vi "Chrg_Dschrg.vi"(3 "Strain Offset":dbl, 4 "PS VISA in":refnum<visa-resource-name>, 5 "PS error in":errorcluster caption="PS error in (no error)", 6 "CyclePath":path=path "C:/Users/ga11/Desktop/VI/results/3PtestCharge.lvm" caption="Filename", 7 "Battery Type":T1(ring), 8 "Charge/discharge":enum8{"Charge", "Discharge"}(ring), 9 "Charge/Discharge Voltage Setpoint":dbl format="%#.6g", 11 "Current Setpoint":dbl format="%#.6g", 13 "Current Cutoff":dbl) -> (14 "PS VISA out":refnum<visa-resource-name>, 16 "Boolean":bool, 19 "PS error out":errorcluster)   [LabVIEW 2020]
uses:
  Drivers-IT-M3400/IT-M3400.lvlib
  <vilib>/Utility/TradDaqScaling.llb/Convert Strain Gauge Reading (scaler).vi
panel:
  out "Read Current(A)":dbl format="%.2g"
  out "Read Voltage(V)":dbl format="%.2g"
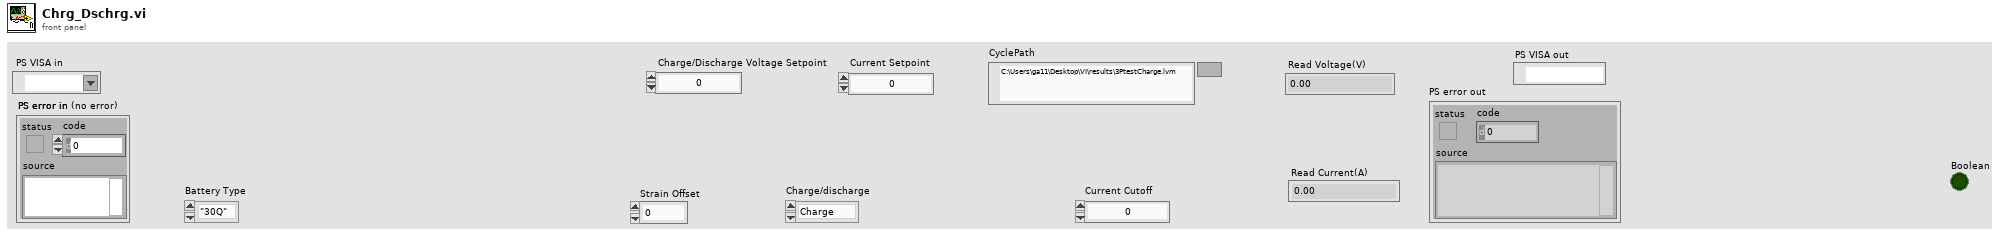
[diagram p1: front panel]
types:
  T1 = enum16{"\"30Q\"", "\"40T\"", "\"2P30Q\"", "\"3P30Q\"", "\"Nissan Leaf\""}
  T2 = cluster{"Baud Rate":u32, "Parity":u16, "Data Bits":u16, "Stop Bits":u16, "Flow Control":u16}
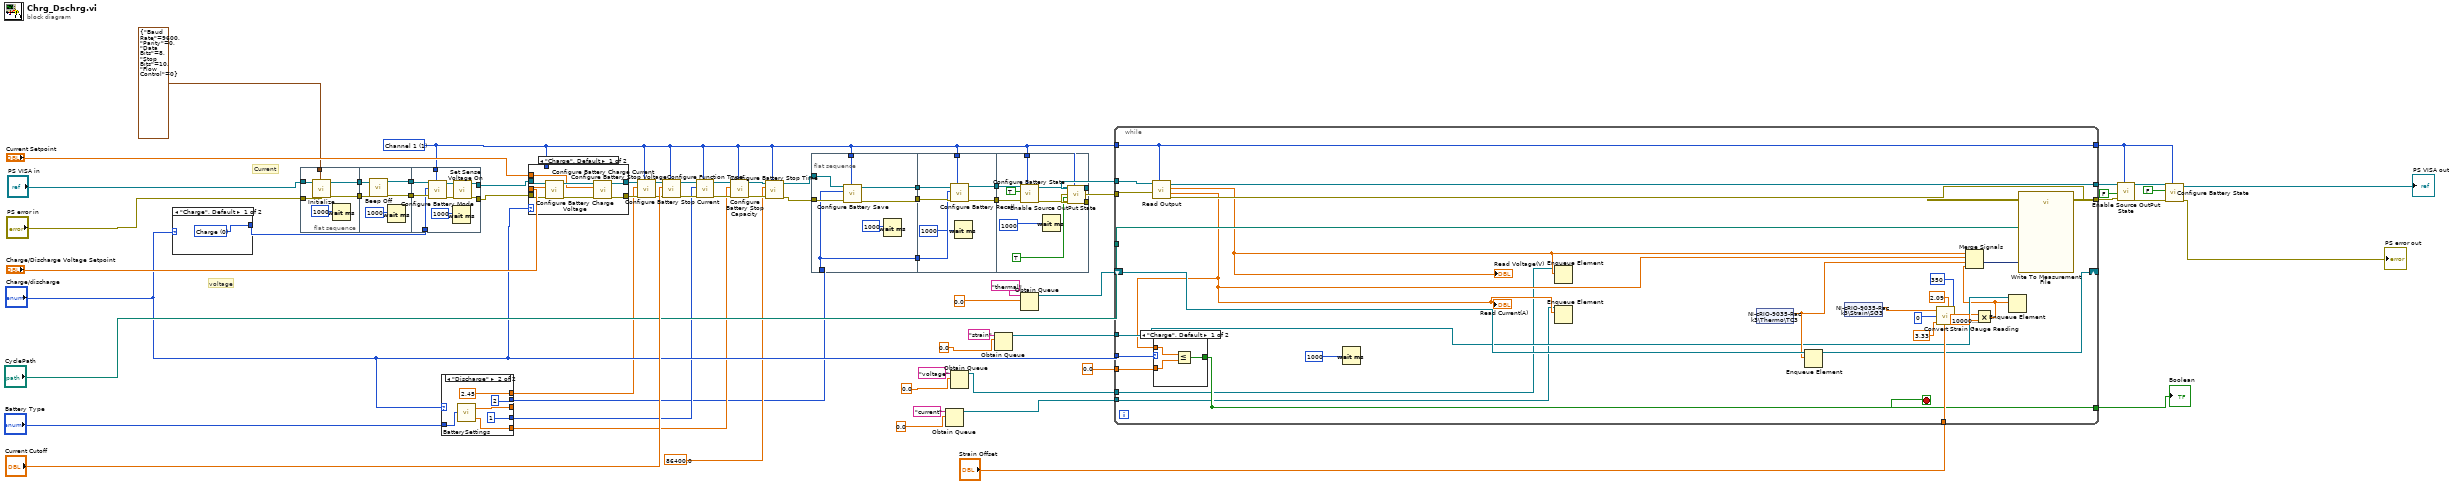
[diagram p0: block diagram]
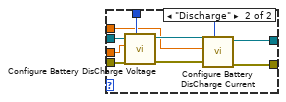
[diagram p2: hidden frame]
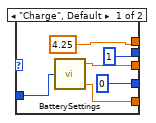
[diagram p3: hidden frame]
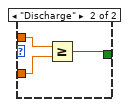
[diagram p4: hidden frame]
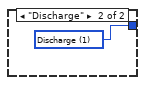
[diagram p5: hidden frame]
diagram:
  w3 = 1 items=["Channel 1"=1, "Channel 2"=2, "Channel 3"=3, "Channel 4"=4, "Channel 5"=5, "Channel 6"=6, "Channel 7"=7, "Channel 8"=8, "Channel 8"=9, "Channel 10"=10, "Channel 11"=11, "Channel 12"=12, "Channel 13"=13, "Channel 14"=14, "Channel 15"=15, "Channel 16"=16] ("Channel")
  # "voltage"
  # "Current"
  n1 = case shown="\"Charge\", Default" "Charge/discharge" {
    tunnel: [w66 w67] -> w6
    frame "Charge", Default {
      w66 = u8 0 items=["Charge", "Discharge"] ("Battery Mode")
    }
    frame "Discharge" {
      w67 = u8 1 items=["Charge", "Discharge"] ("Battery Mode")
    }
  }
  n2 = flat-sequence {
    tunnel: T2 {"Baud Rate"=9600, "Parity"=0, "Data Bits"=8, "Stop Bits"=10, "Flow Control"=0} ("Serial Configuration") -> [w73]
    tunnel: "PS error in" -> [w72]
    tunnel: "PS VISA in" -> [w71]
    tunnel: [w69] -> w11
    tunnel: [w68] -> w10
    tunnel: [w77] -> w9
    tunnel: [w76] -> w8
    tunnel: w11 -> [w75]
    tunnel: w10 -> [w74]
    tunnel: w9 -> [w85]
    tunnel: w8 -> [w86]
    tunnel: w3 -> [w87]
    tunnel: [w80] -> w1
    tunnel: [w81] -> w2
    tunnel: w6 -> [w79]
    frame #0 {
      n3 = call "Initialize.vi"("Serial Configuration"=w73, "error in"=w72, "VISA resource name"=w71) -> ("error out"=w68:errorcluster, "VISA resource name out"=w69:refnum<visa-resource-name>)  [unwired: 7 in]
      n4 = Wait (ms)(milliseconds to wait=1000) -> ()  [unwired: 1 out]
    }
    frame #1 {
      n5 = call "Beep Off.vi"("error in"=w74, "VISA resource name"=w75) -> ("error out"=w76:errorcluster, "VISA resource name out"=w77:refnum<visa-resource-name>)  [unwired: 8 in]
      n6 = Wait (ms)(milliseconds to wait=1000) -> ()  [unwired: 1 out]
    }
    frame #2 {
      n7 = call "Configure Battery Mode.vi"("Channel"=w87, "error in"=w86, "Battery Mode"=w79, "VISA resource name"=w85) -> ("error out"=w82:errorcluster, "VISA resource name out"=w83:refnum<visa-resource-name>)  [unwired: 6 in]
      n8 = Wait (ms)(milliseconds to wait=1000) -> ()  [unwired: 1 out]
      n9 = call "Set Sense Voltage On.vi"("error in"=w82, "VISA resource name"=w83) -> ("error out"=w80:errorcluster, "VISA resource name out"=w81:refnum<visa-resource-name>)  [unwired: 8 in]
    }
  }
  n10 = case shown="\"Discharge\"" "Charge/discharge" {
    tunnel: "Battery Type" -> [w93 w99]
    tunnel: [w92 w97] -> _
    tunnel: [u8 0 ("File") u8 1 ("File")] -> w29
    tunnel: [u8 1 ("File") u8 2 ("File")] -> w27
    tunnel: [w89 w95] -> w28
    tunnel: [4.25 2.45] -> w26
    frame "Charge", Default {
      n11 = call "BatterySettings.vi"("Battery Type"=w93) -> ("RatedCapacity (Ah)"=w89:dbl, "Max Voltage (V)"=w92:dbl)  [unwired: 2 in, 1 out]
    }
    frame "Discharge" {
      n12 = call "BatterySettings.vi"("Battery Type"=w99) -> ("RatedCapacity (Ah)"=w95:dbl, "Min Voltage (V)"=w97:dbl)  [unwired: 2 in, 1 out]
    }
  }
  n13 = case shown="\"Charge\", Default" "Charge/discharge" {
    tunnel: w2 -> [w107 w116]
    tunnel: w1 -> [w106 w115]
    tunnel: [w101 w112] -> w44
    tunnel: [w100 w111] -> w43
    tunnel: w3 -> [_ w110]
    tunnel: "Charge/Discharge Voltage Setpoint" -> [w103 w109]
    tunnel: "Current Setpoint" -> [w102 w108]
    frame "Charge", Default {
      n14 = call "Configure Battery Charge Voltage.vi"("error in"=w106, "Charge Voltage(V)"=w103, "VISA resource name"=w107) -> ("error out"=w104:errorcluster, "VISA resource name out"=w105:refnum<visa-resource-name>)  [unwired: 6 in]
      n15 = call "Configure Battery Charge Current.vi"("error in"=w104, "Charge Current(A)"=w102, "VISA resource name"=w105) -> ("error out"=w100:errorcluster, "VISA resource name out"=w101:refnum<visa-resource-name>)  [unwired: 7 in]
    }
    frame "Discharge" {
      n16 = call "Configure Battery DisCharge Voltage.vi"("Channel"=w110, "error in"=w115, "Discharge Voltage(V)"=w109, "VISA resource name"=w116) -> ("error out"=w113:errorcluster, "VISA resource name out"=w114:refnum<visa-resource-name>)  [unwired: 6 in]
      n17 = call "Configure Battery DisCharge Current.vi"("Channel"=w110, "error in"=w113, "Discharge Current(A)"=w108, "VISA resource name"=w114) -> ("error out"=w111:errorcluster, "VISA resource name out"=w112:refnum<visa-resource-name>)  [unwired: 6 in]
    }
  }
  n18 = call "Configure Battery Stop Voltage.vi"("Channel"=w3, "error in"=w43, "Stop Voltage(V)"=w26, "VISA resource name"=w44) -> ("error out"=w51:errorcluster, "VISA resource name out"=w52:refnum<visa-resource-name>)  [unwired: 6 in]
  n19 = call "Configure Battery Stop Current.vi"("Channel"=w3, "error in"=w51, "Stop Current(A)"="Current Cutoff", "VISA resource name"=w52) -> ("error out"=w31:errorcluster, "VISA resource name out"=w33:refnum<visa-resource-name>)  [unwired: 6 in]
  n20 = call "Configure Function Type.vi"("Channel"=w3, "error in"=w31, "Function Type"=w29, "VISA resource name"=w33) -> ("error out"=w30:errorcluster, "VISA resource name out"=w32:refnum<visa-resource-name>)  [unwired: 6 in]
  n21 = call "Configure Battery Stop Capacity.vi"("Channel"=w3, "error in"=w30, "Stop Capacity(Ah)"=w28, "VISA resource name"=w32) -> ("error out"=w49:errorcluster, "VISA resource name out"=w50:refnum<visa-resource-name>)  [unwired: 6 in]
  n22 = call "Configure Battery Stop Time.vi"("Channel"=w3, "error in"=w49, "Stop Time(S)"=86400.0, "VISA resource name"=w50) -> ("error out"=w35:errorcluster, "VISA resource name out"=w34:refnum<visa-resource-name>)  [unwired: 6 in]
  n23 = flat-sequence {
    tunnel: w27 -> [w122]
    tunnel: w3 -> [w117]
    tunnel: [w120] -> w57
    tunnel: [w122] -> w56
    tunnel: [w119] -> w55
    tunnel: w35 -> [w123]
    tunnel: w34 -> [w121]
    tunnel: [w126] -> w54
    tunnel: [w127] -> w53
    tunnel: w57 -> [w130]
    tunnel: w56 -> [w129]
    tunnel: w55 -> [w128]
    tunnel: w3 -> [w124]
    tunnel: [w134] -> w42
    tunnel: [w133] -> w41
    tunnel: w3 -> [w132]
    tunnel: w54 -> [w140]
    tunnel: w53 -> [w139]
    frame #0 {
      n24 = call "Configure Battery Save.vi"("Channel"=w117, "error in"=w123, "File"=w122, "VISA resource name"=w121) -> ("error out"=w120:errorcluster, "VISA resource name out"=w119:refnum<visa-resource-name>)  [unwired: 6 in]
      n25 = Wait (ms)(milliseconds to wait=1000) -> ()  [unwired: 1 out]
    }
    frame #1 {
      n26 = call "Configure Battery Recall.vi"("Channel"=w124, "error in"=w130, "File"=w129, "VISA resource name"=w128) -> ("error out"=w127:errorcluster, "VISA resource name out"=w126:refnum<visa-resource-name>)  [unwired: 6 in]
      n27 = Wait (ms)(milliseconds to wait=1000) -> ()  [unwired: 1 out]
    }
    frame #2 {
      n28 = call "Configure Battery State.vi"("Channel"=w132, "error in"=w139, "State"=TRUE, "VISA resource name"=w140) -> ("error out"=w137:errorcluster, "VISA resource name out"=w138:refnum<visa-resource-name>)  [unwired: 6 in]
      n29 = Wait (ms)(milliseconds to wait=1000) -> ()  [unwired: 1 out]
      n30 = call "Enable Source OutPut State.vi"("Channel"=w132, "error in"=w137, "State"=TRUE ("Enable Output|Intput"), "VISA resource name"=w138) -> ("error out"=w133:errorcluster, "VISA resource name out"=w134:refnum<visa-resource-name>)  [unwired: 6 in]
    }
  }
  n31 = Obtain Queue(name (unnamed)="current", element data type=0.0) -> (queue out=w16:refnum<queue>)  [unwired: 3 in, 2 out]
  n32 = Obtain Queue(name (unnamed)="voltage", element data type=0.0) -> (queue out=w17:refnum<queue>)  [unwired: 3 in, 2 out]
  n33 = Obtain Queue(name (unnamed)="strain", element data type=0.0) -> (queue out=w20:refnum<queue>)  [unwired: 3 in, 2 out]
  n34 = Obtain Queue(name (unnamed)="thermal", element data type=0.0) -> (queue out=w23:refnum<queue>)  [unwired: 3 in, 2 out]
  n35 = while {
    tunnel: [w161] -> w40
    tunnel: [w159] -> w39
    tunnel: w42 -> [w168]
    tunnel: w41 -> [w167]
    tunnel: w3 -> [w160]
    tunnel: [w160] -> w38
    tunnel: "CyclePath" -> [w165]
    tunnel: 0.0 -> [w163]
    tunnel: "Charge/discharge" -> [w162]
    tunnel: "Strain Offset" -> [w154]
    shift-right: [w150] -> _
    shift-left: w23 -> [w153]
    tunnel: [w151] -> w22
    tunnel: w20 -> [w149]
    tunnel: w17 -> [w142]
    tunnel: w16 -> [w141]
    stop <- w151 stop-if-true
    n36 = call "Read Output.vi"("Channel"=w160, "error in"=w167, "VISA resource name"=w168) -> ("error out"=w159:errorcluster, "Read Current(A)"=w143:dbl, "Read Voltage(V)"=w144:dbl, "VISA resource name out"=w161:refnum<visa-resource-name>)  [unwired: 5 in]
    "Read Voltage(V)" <- w144
    "Read Current(A)" <- w143
    n37 = case shown="\"Charge\", Default" w162 {
      tunnel: w163 -> [w170 w173]
      tunnel: w143 -> [w171 w174]
      tunnel: [w169 w172] -> w151
      frame "Charge", Default {
        n38 = Less Or Equal?(x=w171, y=w170) -> (x <= y?=w169:bool)
      }
      frame "Discharge" {
        n39 = Greater Or Equal?(x=w174, y=w173) -> (x >= y?=w172:bool)
      }
    }
    n40 = Wait (ms)(milliseconds to wait=1000) -> ()  [unwired: 1 out]
    n41 = Enqueue Element(queue=w141, element=w143) -> ()  [unwired: 2 in, 3 out]
    n42 = Enqueue Element(queue=w142, element=w144) -> ()  [unwired: 2 in, 3 out]
    n43 = shared-variable "NI-cRIO-9035-Rack3\\Thermo\\TC3"() -> (w152:dbl)  [unwired: 1 in, 1 out]
    n44 = Enqueue Element(queue=w153, element=w152) -> (queue out=w150:refnum<queue>)  [unwired: 2 in, 2 out]
    n45 = shared-variable "NI-cRIO-9035-Rack3\\Strain\\SG3"() -> (w148:dbl)  [unwired: 1 in, 1 out]
    n46 = call-poly <vilib>:"Convert Strain Gauge Reading.vi"("Vsg (0.0)"=w148, "Bridge Configuration\n(3:Half Bridge II)"=0, "Vex (3.33)"=3.33, "Vinit (0.0)"=w154, "GF (2.0)"=2.09, "Rg (120)"=350) -> ("Strain"=w147:sgl)  [unwired: 4 in]
    n47 = Multiply(x=w147, y=sgl 1000000.0) -> (x*y=w145:sgl)
    n48 = Merge Signals "Merge Signals"(w144, w143, w152, w145) -> (w166:dynamicdata)
    n49 = Enqueue Element(queue=w149, element=w145) -> ()  [unwired: 2 in, 3 out]
    n50 = call "Write To Measurement File"("Signals"=w166, "Filename"=w165) -> ()  [unwired: 15 in, 3 out]
  }
  "Boolean" <- w22
  n51 = call "Enable Source OutPut State.vi"("Channel"=w38, "error in"=w39, "State"=FALSE, "VISA resource name"=w40) -> ("error out"=w47:errorcluster, "VISA resource name out"=w48:refnum<visa-resource-name>)  [unwired: 6 in]
  n52 = call "Configure Battery State.vi"("Channel"=w38, "error in"=w47, "State"=FALSE, "VISA resource name"=w48) -> ("error out"=→"PS error out":errorcluster, "VISA resource name out"=→"PS VISA out":refnum<visa-resource-name>)  [unwired: 6 in]
